vi "DSby2.vi"(11 "Element":cluster{"Older Data":u64, "Newer Data":u64}) -> (3 "Numeric":u64)   [LabVIEW 2020]
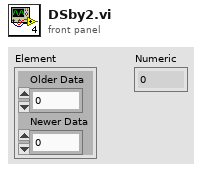
[diagram p1: front panel]
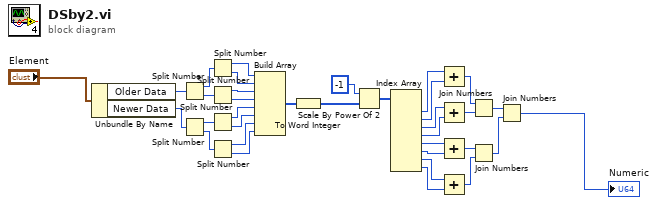
[diagram p0: block diagram]
diagram:
  n1 = Unbundle By Name("Element") -> ("Older Data"=w30:u64, "Newer Data"=w29:u64)
  n2 = Split Number(x=w30) -> (hi(x)=w31:u32, lo(x)=w28:u32)
  n3 = Split Number(x=w29) -> (hi(x)=w27:u32, lo(x)=w26:u32)
  n4 = Split Number(x=w31) -> (hi(x)=w32:u16, lo(x)=w25:u16)
  n5 = Split Number(x=w28) -> (hi(x)=w24:u16, lo(x)=w23:u16)
  n6 = Split Number(x=w27) -> (hi(x)=w22:u16, lo(x)=w21:u16)
  n7 = Split Number(x=w26) -> (hi(x)=w20:u16, lo(x)=w19:u16)
  n8 = Build Array(w32, w25, w24, w23, w22, w21, w20, w19) -> (w18:u16[])
  n9 = To Word Integer(number=w18) -> (16bit integer=w16:i16[])
  n10 = Scale By Power Of 2(n=i16 -1, x=w16) -> (x*2^n=w15:i16[])
  n11 = Index Array(array=w15) -> (element #1=w13:i16, element #2=w14:i16, element #3=w12:i16, element #4=w11:i16, element #5=w10:i16, element #6=w9:i16, element #7=w8:i16, element #8=w7:i16)  [unwired: 8 in]
  n12 = Add(x=w13, y=w14) -> (x+y=w4:i16)
  n13 = Add(x=w12, y=w11) -> (x+y=w3:i16)
  n14 = Add(x=w10, y=w9) -> (x+y=w2:i16)
  n15 = Add(x=w8, y=w7) -> (x+y=w1:i16)
  n16 = Join Numbers(hi=w4, lo=w3) -> ((hi.lo)=w6:u32)
  n17 = Join Numbers(hi=w2, lo=w1) -> ((hi.lo)=w5:u32)
  n18 = Join Numbers(hi=w6, lo=w5) -> ((hi.lo)=→"Numeric":u64)
